vi "Unwrap Barcode.vi"() -> ()   [LabVIEW 2014]
doc: "This example unwraps a circular barcode and reads it."
uses:
  <vilib>/vision/NI_Vision_Development_Module.lvlib
panel:
  out "Unwrapped Image":T1(plugin-control)
  out "Image Source":T1(plugin-control)
  out "Extra Info":T2 {"Barcode Type" items=["Reserved", "Codabar", "Code 39", "Code 93", "Code 128", "EAN 8", "EAN 13", "Interleaved 2 of 5", "MSI", "UPCA"]}
  out "Barcode Result":string
  # "Overview: Demonstrates how to extract and unwrap a region of the image for further processing.\nRequirements: NI Vision Development Module\nInstructions: Run the VI."
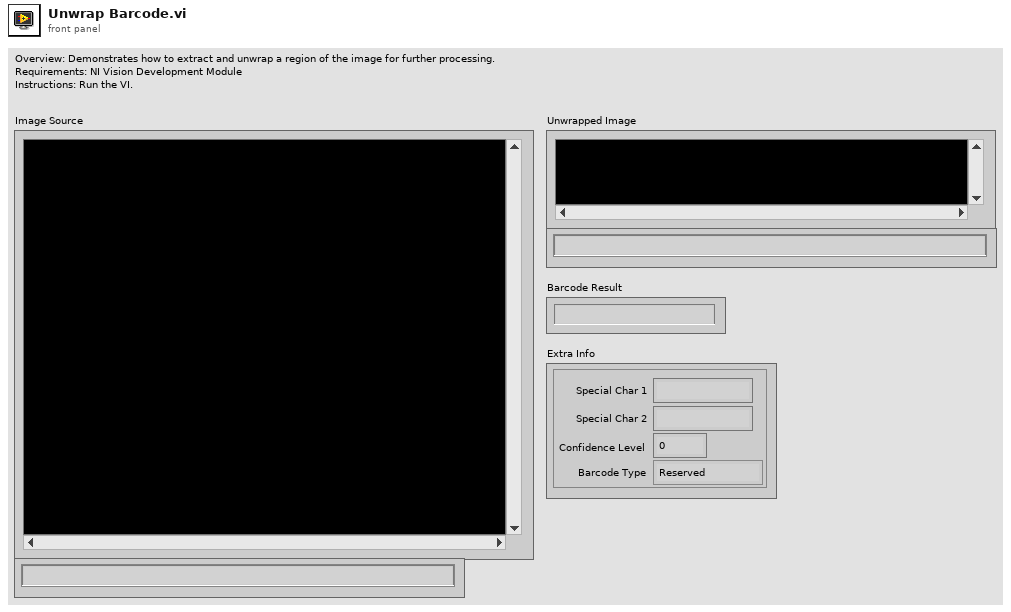
[diagram p1: front panel]
types:
  T1 = typedef "IMAQ Image.ctl" = refnum<image>
  T2 = cluster{"Special Char 1":string, "Special Char 2":string, "Confidence Level":sgl, "Barcode Type":u32}
  T3 = typedef "IMAQ Circle" = cluster{"Center X":i32, "Center Y":i32, "Inner Radius":i32, "Outer Radius":i32, "Start Angle":dbl, "End Angle":dbl}
  T4 = typedef "ROI Descriptor" = cluster{"Global Rectangle":i32[], "Contours":cluster{"ID":enum32{"External", "Internal"}, "Type":u32, "Coordinates":i32[]}[]}
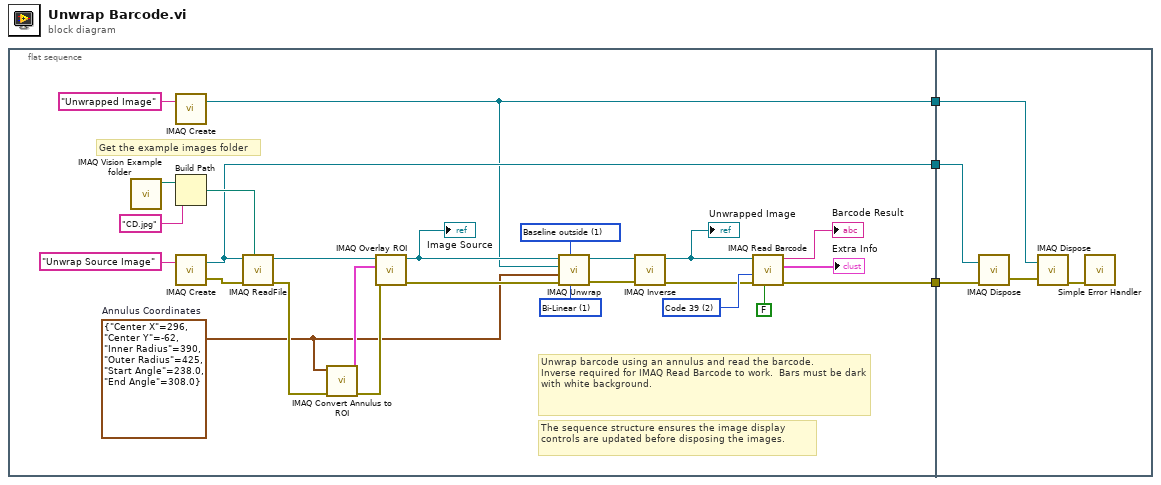
[diagram p0: block diagram]
diagram:
  n1 = flat-sequence {
    tunnel: [w10] -> w3
    tunnel: [w5] -> w2
    tunnel: [w6] -> w1
    tunnel: w3 -> [w34]
    tunnel: w2 -> [w30]
    tunnel: w1 -> [w31]
    frame #0 {
      w4 = T3 {"Center X"=296, "Center Y"=-62, "Inner Radius"=390, "Outer Radius"=425, "Start Angle"=238.0, "End Angle"=308.0}  # Annulus Coordinates
      w16 = u32 1 items=["Baseline inside", "Baseline outside"] ("Text Orientation")
      w17 = u32 1 items=["Zero Order", "Bi-Linear", "Quadratic", "Cubic Spline"] ("Interpolation Type")
      w21 = u32 2 items=["Reserved", "Codabar", "Code 39", "Code 93", "Code 128", "EAN 8", "EAN 13", "Interleaved 2 of 5", "MSI", "UPCA"] ("Barcode Type")
      # "The sequence structure ensures the image display controls are updated before disposing the images."
      # "Unwrap barcode using an annulus and read the barcode.\nInverse required for IMAQ Read Barcode to work.  Bars must be dark with white background."
      # "Get the example images folder"
      n2 = call "IMAQ Vision Example folder.vi"() -> ("Example Image Path"=w29:path)  [unwired: 11 in]
      n3 = call "IMAQ Create"("Image Name"="Unwrapped Image") -> ("New Image"=w5:T1)  [unwired: 4 in, 1 out]
      n4 = Build Path(base path=w29, name or relative path="CD.jpg") -> (appended path=w27:path)
      n5 = call "IMAQ Create"("Image Name"="Unwrap Source Image") -> ("New Image"=w6:T1, "error out"=w25:errorcluster)  [unwired: 4 in]
      n6 = call "IMAQ ReadFile"("File Path"=w27, "error in (no error)"=w25, "Image"=w6) -> ("error out"=w12:errorcluster, "Image Out"=w7:T1)  [unwired: 4 in, 3 out]
      n7 = call "IMAQ Convert Annulus to ROI"("error in (no error)"=w12, "Annulus"=w4) -> ("error out"=w22:errorcluster, "ROI Descriptor"=w23:T4)  [unwired: 7 in]
      n8 = call "IMAQ Overlay ROI"("error in (no error)"=w22, "ROI Descriptor"=w23, "Image"=w7) -> ("error out"=w11:errorcluster, "Image Out"=w8:T1)  [unwired: 7 in]
      "Image Source" <- w8
      n9 = call "IMAQ Unwrap"("Image Src"=w8, "Orientation"=w16, "Image Dst"=w5, "Annulus"=w4, "Interpolation Type"=w17, "error in (no error)"=w11) -> ("Image Dst Out"=w13:T1, "error out"=w15:errorcluster)  [unwired: 1 in]
      n10 = call "IMAQ Inverse"("error in (no error)"=w15, "Image Src"=w13) -> ("error out"=w14:errorcluster, "Image Dst Out"=w9:T1)  [unwired: 8 in]
      "Unwrapped Image" <- w9
      n11 = call "IMAQ Read Barcode"("Validate"=FALSE, "error in (no error)"=w14, "Barcode Type"=w21, "Image"=w9) -> ("error out"=w10:errorcluster, "Extra Info"=→"Extra Info":T2, "String"=→"Barcode Result":string)  [unwired: 4 in, 1 out]
    }
    frame #1 {
      n12 = call "IMAQ Dispose"("Image"=w31, "error in (no error)"=w34) -> ("error out"=w33:errorcluster)  [unwired: 4 in]
      n13 = call "IMAQ Dispose"("Image"=w30, "error in (no error)"=w33) -> ("error out"=w32:errorcluster)  [unwired: 4 in]
      n14 = call <vilib>:"Simple Error Handler.vi"("error in (no error)"=w32) -> ()  [unwired: 4 in, 5 out]
    }
  }
